vi "Tap Once.vi"(8 "error in (no error)":errorcluster, 11 "Call time (s)":dbl) -> (0 "error out":errorcluster)   [LabVIEW 2014]
uses:
  Globals.vi
  <vilib>/LabVIEW Hacker/LINX/Public/Peripherals/Digital/Digital Write 1 Chan.vi
  <vilib>/LabVIEW Hacker/LINX/LVH-LINX.lvlib
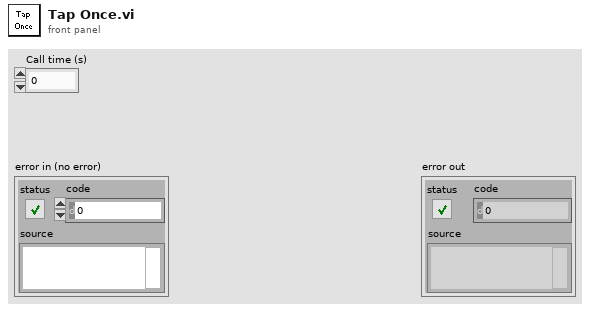
[diagram p1: front panel]
types:
  T1 = typedef "LVH-LINX.lvlib/LINX Ref.ctl" = cluster{"Platform":T2, "Interface":T3, "LINX Device Config":T4}
  T2 = typedef "LVH-LINX.lvlib/Platform.ctl" = enum16{"LINX", "myRIO"}
  T3 = typedef "LVH-LINX.lvlib/Interface.ctl" = enum16{"Serial", "TCP"}
  T4 = typedef "LVH-LINX.lvlib/Device.lvlib/LINX Device Config.ctl" = cluster{"Interface":T3, "COM Port":refnum<visa-resource-name>, "TCP Configuration":T5, "Device Family":T6, "Device ID":u8, "Device Name":string, "TCP Ref":refnum<k5>}
  T5 = typedef "LVH-LINX.lvlib/Device.lvlib/TCP Config.ctl" = cluster{"IP Address":string, "Port":u16}
  T6 = typedef "LVH-LINX.lvlib/Device Family.ctl" = enum8{"National Instruments", "Digilent", "Arduino"}
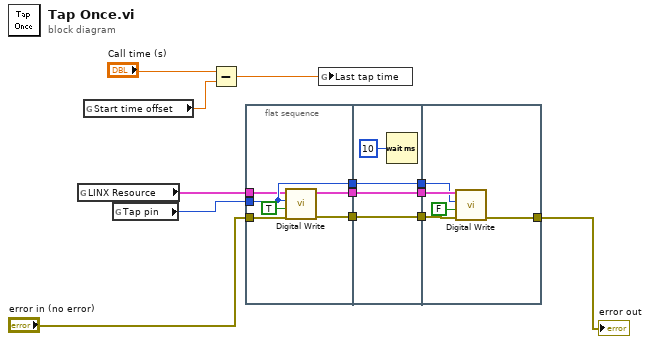
[diagram p0: block diagram]
diagram:
  n1 = global read "Globals.vi" "LINX Resource"() -> (w6:T1)
  n2 = global read "Globals.vi" "Start time offset"() -> (w8:dbl)
  n3 = global read "Globals.vi" "Tap pin"() -> (w7:u32)
  n4 = Subtract(x="Call time (s)", y=w8) -> (x-y=w9:dbl)
  n5 = flat-sequence {
    tunnel: [w18] -> w13
    tunnel: w7 -> [w17]
    tunnel: [w17] -> w12
    tunnel: w6 -> [w16]
    tunnel: "error in (no error)" -> [w15]
    tunnel: [w14] -> w2
    tunnel: [w22] -> w11
    tunnel: w13 -> [w22]
    tunnel: [w21] -> w10
    tunnel: w12 -> [w21]
    tunnel: [w20] -> w3
    tunnel: w2 -> [w20]
    tunnel: w11 -> [w27]
    tunnel: w10 -> [w26]
    tunnel: w3 -> [w25]
    tunnel: [w24] -> w1
    frame #0 {
      n6 = call-poly <vilib>:"Digital Write.vi"("Error In"=w15, "Output Value"=TRUE, "DO Channel"=w17, "LINX Resource"=w16) -> ("Error Out"=w14:errorcluster, "LINX Resource"=w18:T1)  [unwired: 6 in]
    }
    frame #1 {
      n7 = Wait (ms)(milliseconds to wait=u32 10) -> ()  [unwired: 1 out]
    }
    frame #2 {
      n8 = call-poly <vilib>:"Digital Write.vi"("Error In"=w25, "Output Value"=FALSE, "DO Channel"=w26, "LINX Resource"=w27) -> ("Error Out"=w24:errorcluster)  [unwired: 6 in, 1 out]
    }
  }
  n9 = global write "Globals.vi" "Last tap time"(w9) -> ()
  "error out" <- w1
